vi "Thermal Chamber Controller_DQMH_Action Update Heater State-teardown.vi"(8 "error in (no error)":errorcluster, 11 "test case ID":string) -> (3 "result":bool)   [LabVIEW 2018]
doc: "The teardown VI should be executed after the VI under test in the harness VI. In this VI you can evaluate the outputs of the VI under test.\n\nSee the Help Document for more information. (<b>Help</b> > <b>IncQuery Labs</b> > <b>InstaCoverage</b> > <b>InstaCoverage Help...</b>)"
uses:
  Libraries/Thermal Chamber Response Simulator/Thermal Chamber Response Simulator.lvlib
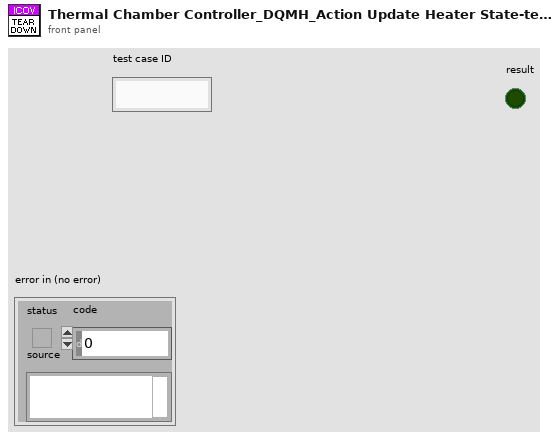
[diagram p1: front panel]
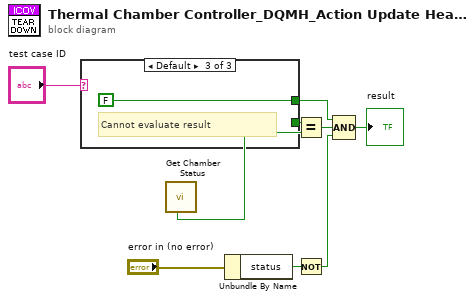
[diagram p0: block diagram]
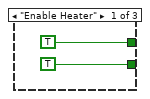
[diagram p2: hidden frame]
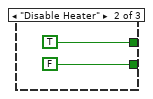
[diagram p3: hidden frame]
diagram:
  n1 = case shown="Default" "test case ID" {
    tunnel: [TRUE ("Heater State") FALSE ("Heater State") _] -> w7
    tunnel: [TRUE ("value") TRUE ("value") FALSE ("value")] -> w5
    frame "Enable Heater" {
    }
    frame "Disable Heater" {
    }
    frame Default {
      # "Cannot evaluate result"
    }
  }
  n2 = call "Get Chamber Status.vi"() -> ("Heater State"=w6:bool)  [unwired: 6 in, 5 out]
  n3 = Unbundle By Name("error in (no error)") -> ("status"=w3:bool)
  n4 = Equal?(x=w7, y=w6) -> (x = y?=w9:bool)
  n5 = Not(x=w3) -> (.not. x?=w2:bool)
  n6 = Compound Arithmetic op=AND(w5, w9, w2) -> (→"result":bool)
